vi "Get All Names and Values.vi"(8 "error in (no error)":errorcluster, 11 "LUT in":refnum<class "LUT.lvclass">) -> (0 "error out":errorcluster, 1 "Values":variant[](array[variant]), 2 "Names":string[](array[string]), 3 "LUT out":refnum<class "LUT.lvclass">)   [LabVIEW 2017, in "LUT.lvlib" / "LUT.lvclass"]
doc: "Returns the names of all attributes and their corresponding values in 1D arrays."
uses:
  LUT.lvclass
  LUT.lvclass/LUT.ctl
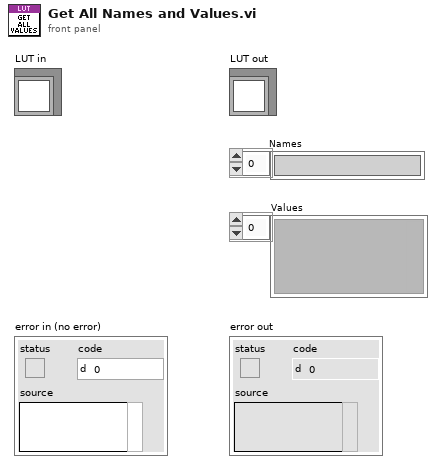
[diagram p1: front panel]
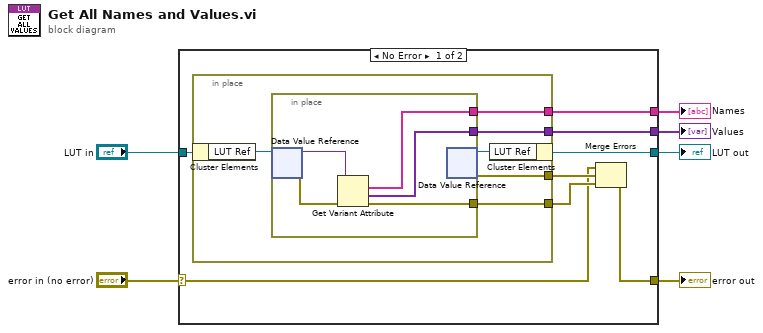
[diagram p0: block diagram]
diagram:
  n1 = case shown="No Error" "error in (no error)" {
    selector: "error in (no error)" -> [w8 w27]
    tunnel: [w7 w27] -> w5
    tunnel: [w13 w26] -> w3
    tunnel: "LUT in" -> [w14 w26]
    tunnel: [w12 _] -> w1
    tunnel: [w11 _] -> w2
    frame No Error {
      n2 = in-place {
        in-place-border: [w18] -> w12
        in-place-border: [w17] -> w11
        in-place-border: [w16] -> w9
        in-place-border: [w15] -> w10
        n3 = in-place-cluster #1(w14) -> ("LUT Ref"=w20:refnum<data-value>)
        n4 = in-place {
          in-place-border: [w25] -> w18
          in-place-border: [w24] -> w17
          in-place-border: [w22] -> w16
          n5 = in-place-dvr #2(w20) -> (w21:variant, w23:errorcluster)
          n6 = Get Variant Attribute(Variant=w21, error in=w23) -> (names=w24:string[], values=w25:variant[], error out=w22:errorcluster)  [unwired: 2 in, 1 out]
          n7 = in-place-dvr #2() -> (w19:refnum<data-value>, w15:errorcluster)  [unwired: 1 in]
        }
        n8 = in-place-cluster #1("LUT Ref"=w19) -> (w13:refnum<class "LUT.lvclass">)
      }
      n9 = Merge Errors(w8, w10, w9) -> (w7:errorcluster)
    }
    frame Error {
    }
  }
  "error out" <- w5
  "LUT out" <- w3
  "Values" <- w1
  "Names" <- w2
